vi "ActionVIOnCompile.vi"(8 "error in (no error)":errorcluster, 11 "Device Item Ref in":T1 format="%.0x") -> (0 "error out":errorcluster)   [LabVIEW 2017, in "Chassis TimeSync System Explorer.lvlib"]
uses:
  Chassis TimeSync System Explorer.lvlib
  <vilib>/NI Veristand/Custom Device API/Custom Device Item Ref.ctl
  Shared/Compiled Data.ctl
  Shared/Connection Settings.ctl
  Shared/Mode.ctl
  Shared/External Pin.ctl
  Shared/Routes.ctl
  Shared/Route.ctl
  Shared/Time Ref Settings.ctl
  Shared/Time Reference.ctl
  Shared/IRIG Type.ctl
  ClockTrigger_routing.ctl
  Shared/Constants.vi
  <vilib>/NI Veristand/Custom Device API/Get Item Property (String).vi
  <vilib>/NI Veristand/Custom Device API/Get Item Property (U16).vi
  <vilib>/NI Veristand/Custom Device API/Get Item Property (Double).vi
  <vilib>/NI Veristand/Custom Device API/Get Item Property (Boolean).vi
  <vilib>/NI Veristand/Custom Device API/Get Item Property (Variant).vi
  <vilib>/NI Veristand/Custom Device API/Set Item Property (Variant).vi
  Shared/Chassis TimeSync Shared.lvlib
  <vilib>/NI Veristand/Custom Device API/Custom Device API.lvlib
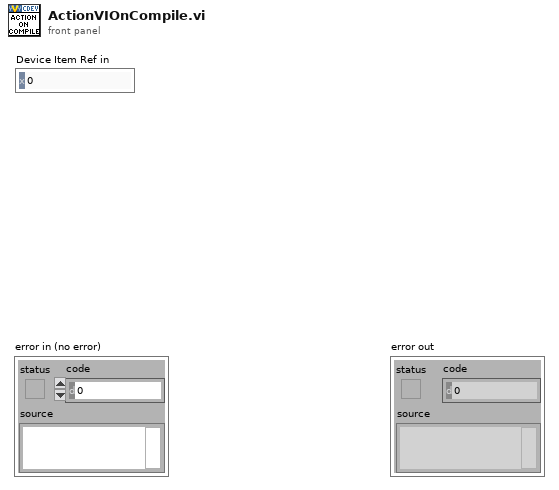
[diagram p1: front panel]
types:
  T1 = typedef "Custom Device API.lvlib/Custom Device Item Ref.ctl" = u64
  T2 = typedef "Chassis TimeSync System Explorer.lvlib/ClockTrigger_routing.ctl" = cluster{"Shared Trigger Source Terminal (Master Chassis)":string, "Master Trigger Output":string, "Export Clock":bool, "Export Trigger":bool}
  T3 = typedef "Chassis TimeSync Shared.lvlib/Compiled Data.ctl" = cluster{"SyncMod?":bool, "SyncMod":string, "ConnectionSettings":T4, "TimeKeeper":string, "ScanOffset(%)":dbl, "StartDelay(s)":u16, "Time Ref Settings":T9, "FIFO Locations":cluster{"SysTime":i32[], "TimeRef":i32[], "Status":i32[]}, "Clock and Trigger Routing":T2}
  T4 = typedef "Chassis TimeSync Shared.lvlib/Connection Settings.ctl" = cluster{"Mode":T5, "pxitrig":bool, "pfi0":bool, "pfi1":bool, "pfi2":bool, "External Pin":T6, "Routes":T7, "pxitrig1_ts":bool}
  T5 = typedef "Chassis TimeSync Shared.lvlib/Mode.ctl" = enum16{"Generate sample clock", "Route sample clock out of chassis", "Route sample clock into chassis", "Custom routes"}
  T6 = typedef "Chassis TimeSync Shared.lvlib/External Pin.ctl" = enum16{"PFI0", "PFI1", "PFI2"}
  T7 = typedef "Chassis TimeSync Shared.lvlib/Routes.ctl" = T8[]
  T8 = typedef "Chassis TimeSync Shared.lvlib/Route.ctl" = cluster{"Source":string, "Destination":string}
  T9 = typedef "Chassis TimeSync Shared.lvlib/Time Ref Settings.ctl" = cluster{"Time Reference":T10, "Priority 1":i32, "Priority 2":i32, "IRIG type":T11, "Terminal":string, "PPSSetTime":bool, "Start Time":timestamp}
  T10 = typedef "Chassis TimeSync Shared.lvlib/Time Reference.ctl" = enum16{"GPS", "IRIG", "PPS", "1588 Ordinary Clock", "PXI Chassis Clock", "Free Running (Internal)"}
  T11 = typedef "Chassis TimeSync Shared.lvlib/IRIG Type.ctl" = enum16{"IRIGB DC", "IRIGB AM"}
  T12 = typedef "Chassis TimeSync Shared.lvlib/Channel.ctl" = cluster{"Name":string, "Units":string, "Default":dbl, "Description":string}
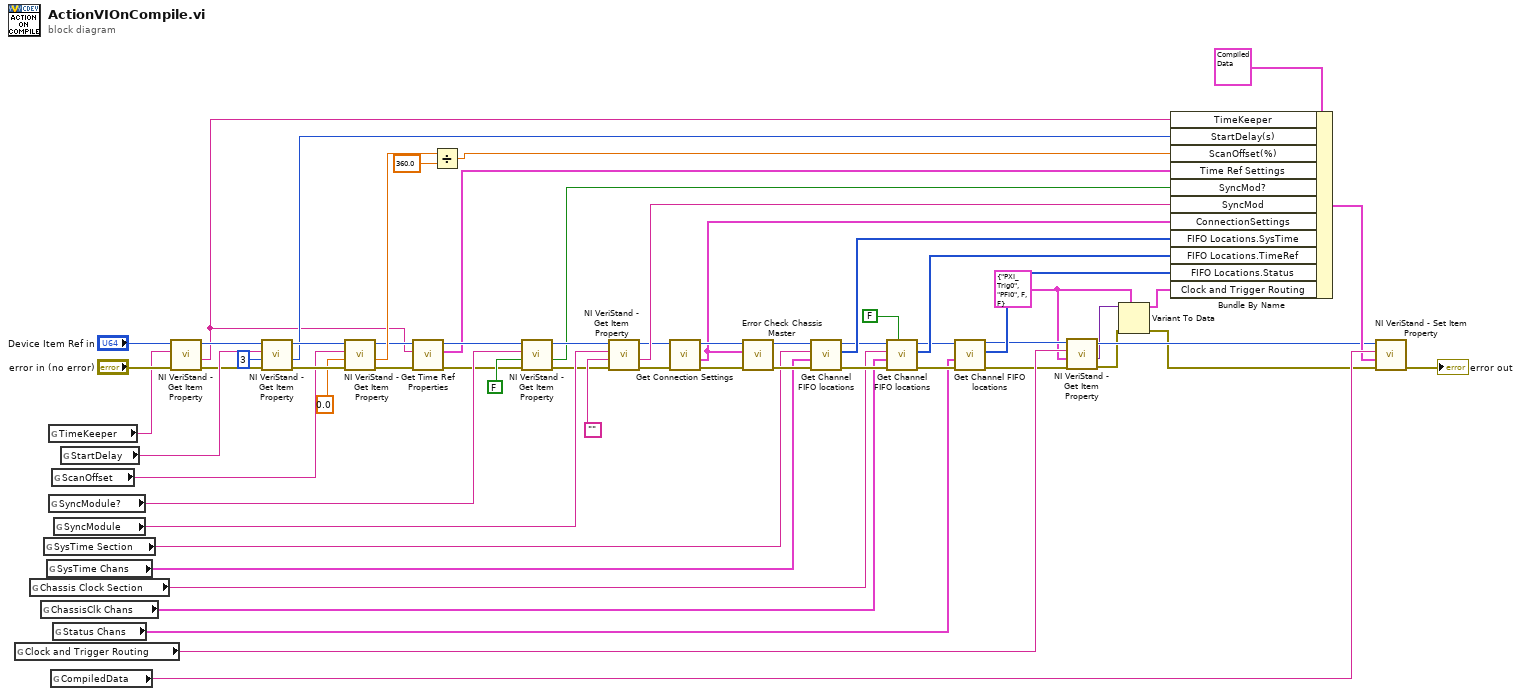
[diagram p0: block diagram]
diagram:
  w1 = T2 {"Shared Trigger Source Terminal (Master Chassis)"="PXI_Trig0", "Master Trigger Output"="PFI0", "Export Clock"=FALSE, "Export Trigger"=FALSE} ("Clock and Trigger Routing")
  n1 = global read "Constants.vi" "Clock and Trigger Routing"() -> (w9:string)
  n2 = global read "Constants.vi" "Chassis Clock Section"() -> (w18:string)
  n3 = global read "Constants.vi" "ChassisClk Chans"() -> (w17:T12[])
  n4 = global read "Constants.vi" "SysTime Section"() -> (w22:string)
  n5 = global read "Constants.vi" "SysTime Chans"() -> (w23:T12[])
  n6 = global read "Constants.vi" "TimeKeeper"() -> (w60:string)
  n7 = global read "Constants.vi" "SyncModule?"() -> (w44:string)
  n8 = global read "Constants.vi" "CompiledData"() -> (w27:string)
  n9 = global read "Constants.vi" "ScanOffset"() -> (w55:string)
  n10 = global read "Constants.vi" "Status Chans"() -> (w13:T12[])
  n11 = global read "Constants.vi" "SyncModule"() -> (w42:string)
  n12 = global read "Constants.vi" "StartDelay"() -> (w57:string)
  n13 = call-poly <vilib>:"NI VeriStand - Get Item Property.vi"("error in (no error)"="error in (no error)", "Property Name"=w60, "Item Ref in"="Device Item Ref in") -> ("error out"=w53:errorcluster, "Value"=w45:string, "Item Ref out"=w52:T1)  [unwired: 5 in, 1 out]
  n14 = call-poly <vilib>:"NI VeriStand - Get Item Property.vi"("error in (no error)"=w53, "Default Value"=u16 3 ("Start Offset Multiple"), "Property Name"=w57, "Item Ref in"=w52) -> ("error out"=w58:errorcluster, "Value"=w51:u16, "Item Ref out"=w59:T1)  [unwired: 4 in, 1 out]
  n15 = call-poly <vilib>:"NI VeriStand - Get Item Property.vi"("error in (no error)"=w58, "Default Value"=0.0 ("Scan Offset Scale (%)"), "Property Name"=w55, "Item Ref in"=w59) -> ("error out"=w47:errorcluster, "Value"=w50:dbl, "Item Ref out"=w46:T1)  [unwired: 4 in, 1 out]
  n16 = call "Get Time Ref Properties.vi"("error in (no error)"=w47, "TimeKeeper Module"=w45, "Device Item Ref in"=w46) -> ("error out"=w40:errorcluster, "Time Ref Settings"=w33:T9, "Item Ref out"=w39:T1)  [unwired: 6 in]
  n17 = Divide(x=w50, y=360.0) -> (x/y=w49:dbl)
  n18 = call-poly <vilib>:"NI VeriStand - Get Item Property.vi"("error in (no error)"=w40, "Default Value"=FALSE, "Property Name"=w44, "Item Ref in"=w39) -> ("error out"=w37:errorcluster, "Value"=w36:bool, "Item Ref out"=w38:T1)  [unwired: 4 in, 1 out]
  n19 = call-poly <vilib>:"NI VeriStand - Get Item Property.vi"("error in (no error)"=w37, "Default Value"="", "Property Name"=w42, "Item Ref in"=w38) -> ("error out"=w34:errorcluster, "Value"=w35:string, "Item Ref out"=w31:T1)  [unwired: 4 in, 1 out]
  n20 = call "Get Connection Settings.vi"("error in (no error)"=w34, "Item Ref in"=w31) -> ("error out"=w32:errorcluster, "Connection Settings"=w29:T4, "Item Ref out"=w30:T1)  [unwired: 6 in, 1 out]
  n21 = call "Error Check Chassis Master.vi"("error in (no error)"=w32, "Connection Settings"=w29, "Item Ref in"=w30) -> ("error out"=w25:errorcluster, "Item Ref out"=w24:T1)  [unwired: 7 in]
  n22 = call "Get Channel FIFO locations.vi"("error in (no error)"=w25, "Channels to get refs"=w23, "Section By Relative Path (\"\")"=w22, "Device Ref in"=w24) -> ("error out"=w20:errorcluster, "FIFO Locations"=w21:i32[], "Device Ref out"=w19:T1)  [unwired: 5 in]
  n23 = call "Get Channel FIFO locations.vi"("Error On Missing Section? (T)"=FALSE, "error in (no error)"=w20, "Channels to get refs"=w17, "Section By Relative Path (\"\")"=w18, "Device Ref in"=w19) -> ("error out"=w15:errorcluster, "FIFO Locations"=w16:i32[], "Device Ref out"=w14:T1)  [unwired: 4 in]
  n24 = call "Get Channel FIFO locations.vi"("error in (no error)"=w15, "Channels to get refs"=w13, "Device Ref in"=w14) -> ("error out"=w7:errorcluster, "FIFO Locations"=w12:i32[], "Device Ref out"=w8:T1)  [unwired: 6 in]
  n25 = call-poly <vilib>:"NI VeriStand - Get Item Property.vi"("error in (no error)"=w7, "Default Value"=w1, "Property Name"=w9, "Item Ref in"=w8) -> ("error out"=w5:errorcluster, "Value"=w4:variant, "Item Ref out"=w6:T1)  [unwired: 4 in, 1 out]
  n26 = Variant To Data(error in=w5, type=w1, Variant=w4) -> (data=w3:T2, error out=w2:errorcluster)
  n27 = Bundle By Name(cluster=T3 {"SyncMod?"=FALSE, "SyncMod"="", "ConnectionSettings"={"Mode"=enum."Generate sample clock", "pxitrig"=FALSE, "pfi0"=FALSE, "pfi1"=FALSE, "pfi2"=FALSE, "External Pin"=enum."PFI0", "Routes"=[], "pxitrig1_ts"=FALSE}, "TimeKeeper"="", "ScanOffset(%)"=0.0, "StartDelay(s)"=0, "Time Ref Settings"={"Time Reference"=enum."GPS", "Priority 1"=0, "Priority 2"=0, "IRIG type"=enum."IRIGB AM", "Terminal"="", "PPSSetTime"=FALSE, "Start Time"=timestamp(0 s since 1904-01-01)}, "FIFO Locations"={"SysTime"=[], "TimeRef"=[], "Status"=[]}, "Clock and Trigger Routing"={"Shared Trigger Source Terminal (Master Chassis)"="PXI_Trig0", "Master Trigger Output"="PFI0", "Export Clock"=FALSE, "Export Trigger"=FALSE}} ("Compiled Data"), "TimeKeeper"=w45, "StartDelay(s)"=w51, "ScanOffset(%)"=w49, "Time Ref Settings"=w33, "SyncMod?"=w36, "SyncMod"=w35, "ConnectionSettings"=w29, "FIFO Locations.SysTime"=w21, "FIFO Locations.TimeRef"=w16, "FIFO Locations.Status"=w12, "Clock and Trigger Routing"=w3) -> (w26:T3)
  n28 = call-poly <vilib>:"NI VeriStand - Set Item Property.vi"("error in (no error)"=w2, "Value"=w26, "Property Name"=w27, "Item Ref in"=w6) -> ("error out"=→"error out":errorcluster)  [unwired: 5 in, 2 out]
